vi "Deviated Result.vi"(8 "Error in":errorcluster, 11 "ADC in":refnum<class "ADC.lvclass">) -> (0 "Error out":errorcluster, 3 "ADC out":refnum<class "ADC.lvclass">)   [LabVIEW 2020, in "ADC.lvclass"]
doc: "Generates deviated values for ADC"
uses:
  ADC.lvclass
  C:/Users/kavin.palanisamy/Downloads/SDLC Sample updated/SDLC/Builds/Source Distribution/Device/Device.lvclass
  <vilib>/numeric/Random Number (Range) DBL.vi
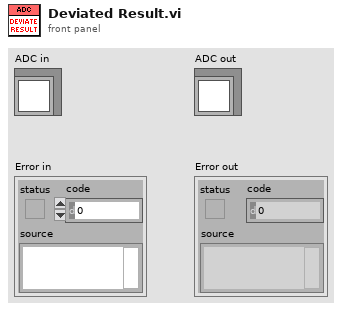
[diagram p1: front panel]
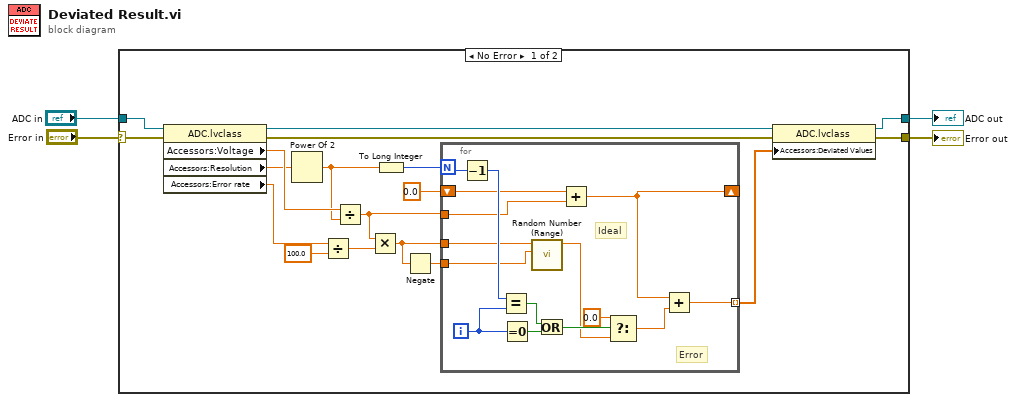
[diagram p0: block diagram]
diagram:
  n1 = case shown="No Error" "Error in" {
    selector: "Error in" -> [w22 w38]
    tunnel: "ADC in" -> [w21 w39]
    tunnel: [w12 w38] -> w2
    tunnel: [w11 w39] -> w1
    frame No Error {
      n2 = property class="ADC.lvclass"(reference=w21, error in=w22) -> (reference out=w13:refnum<class "ADC.lvclass">, error out=w14:errorcluster, "Accessors:Voltage"=w20:dbl, "Accessors:Resolution"=w19:dbl, "Accessors:Error rate"=w17:dbl)
      n3 = Power Of 2(x=w19) -> (2^x=w8:dbl)
      n4 = Divide(x=w17, y=100.0) -> (x/y=w15:dbl)
      n5 = Divide(x=w20, y=w8) -> (x/y=w7:dbl)
      n6 = Multiply(x=w7, y=w15) -> (x*y=w9:dbl)
      n7 = To Long Integer(number=w8) -> (32bit integer=w18:i32)
      n8 = Negate(x=w9) -> (-x=w10:dbl)
      n9 = for {
        N: w18 -> [w35]
        tunnel: w9 -> [w31]
        tunnel: w10 -> [w29]
        tunnel: w7 -> [w28]
        shift-right: [w25] -> _
        shift-left: 0.0 ("x") -> [w27]
        tunnel: [w24] -> w5 mode=indexing
        i -> [w36]
        # "Error"
        # "Ideal"
        n10 = Decrement(x=w35) -> (x-1=w34:i32)
        n11 = Equal?(x=w34, y=w36) -> (x = y?=w33:bool)
        n12 = Equal To 0?(x=w36) -> (x = 0?=w37:bool)
        n13 = call-poly <vilib>:"Random Number (Range).vi"("lower bound (0)"=w29, "upper bound (100)"=w31) -> ("number"=w23:dbl)  [unwired: 9 in]
        n14 = Or(x=w33, y=w37) -> (x .or. y?=w32:bool)
        n15 = Add(x=w27, y=w28) -> (x+y=w25:dbl)
        n16 = Select(t=0.0, s=w32, f=w23) -> (s? t:f=w26:dbl)
        n17 = Add(x=w25, y=w26) -> (x+y=w24:dbl)
      }
      n18 = property class="ADC.lvclass"(reference=w13, error in=w14, "Accessors:Deviated Values"=w5) -> (reference out=w11:refnum<class "ADC.lvclass">, error out=w12:errorcluster)
    }
    frame Error {
    }
  }
  "Error out" <- w2
  "ADC out" <- w1
